vi "Variant to String.vi"(8 "error in (no error)":errorcluster, 10 "datatype":T1, 11 "Variant":variant) -> (0 "error out":errorcluster, 3 "String":string)   [LabVIEW 2016, in "DataGrid.lvlib" / "DataTable.lvclass"]
uses:
  <userlib>/LabVIEWdotNetDataGrid/source/DataTable/DataTable.lvclass
  <userlib>/LabVIEWdotNetDataGrid/source/GridColumn/ColumnType.ctl
  <userlib>/LabVIEWdotNetDataGrid/source/GridColumn/GridColumn.lvclass
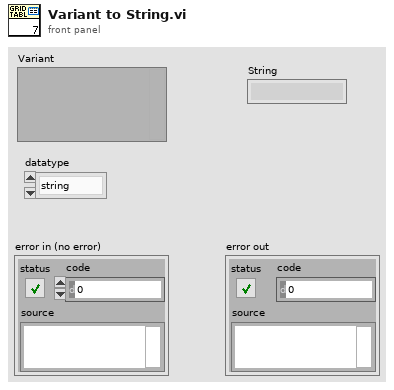
[diagram p1: front panel]
types:
  T1 = typedef "DataGrid.lvlib/GridColumn.lvclass/ColumnType.ctl" = enum16{"string", "image", "check", "numeric", "timestamp", "button", "combo", "link"}
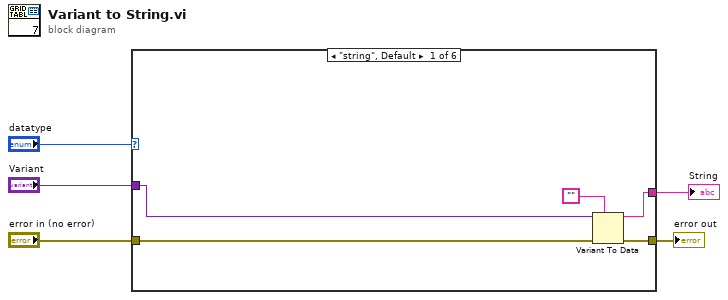
[diagram p0: block diagram]
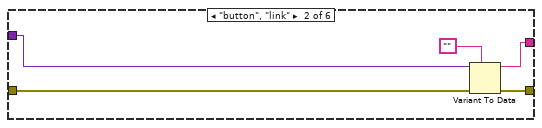
[diagram p2: hidden frame]
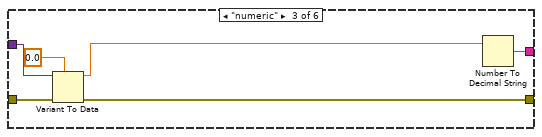
[diagram p3: hidden frame]
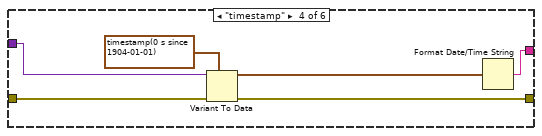
[diagram p4: hidden frame]
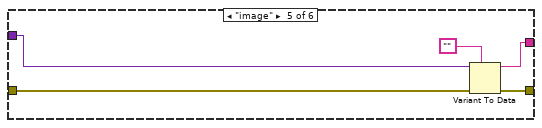
[diagram p5: hidden frame]
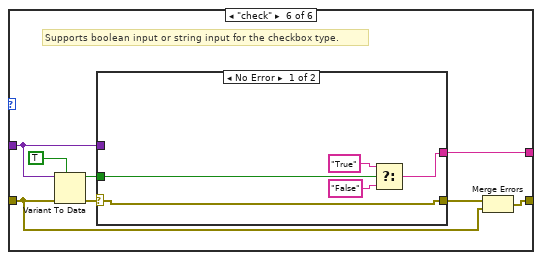
[diagram p6: hidden frame]
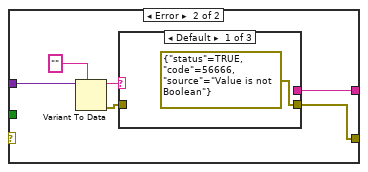
[diagram p7: hidden frame]
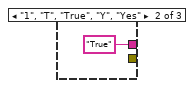
[diagram p8: hidden frame]
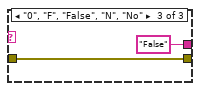
[diagram p9: hidden frame]
diagram:
  n1 = case shown="\"string\", Default" "datatype" {
    tunnel: "Variant" -> [w9 w14 w21 w27 w31 w37]
    tunnel: "error in (no error)" -> [w10 w15 w17 w23 w32 w35]
    tunnel: [w6 w11 w16 w22 w28 w34] -> w4
    tunnel: [w7 w12 w18 w24 w29 w33] -> w1
    frame "string", Default {
      n2 = Variant To Data(error in=w10, type="", Variant=w9) -> (data=w7:string, error out=w6:errorcluster)
    }
    frame "button", "link" {
      n3 = Variant To Data(error in=w15, type="", Variant=w14) -> (data=w12:string, error out=w11:errorcluster)
    }
    frame "numeric" {
      n4 = Variant To Data(error in=w17, type=0.0, Variant=w21) -> (data=w19:dbl, error out=w16:errorcluster)
      n5 = Number To Decimal String(number=w19) -> (decimal integer string=w18:string)  [unwired: 1 in]
    }
    frame "timestamp" {
      n6 = Variant To Data(error in=w23, type=timestamp(0 s since 1904-01-01), Variant=w27) -> (data=w25:timestamp, error out=w22:errorcluster)
      n7 = Format Date/Time String(seconds (now)=w25) -> (date/time string=w24:string)  [unwired: 2 in]
    }
    frame "image" {
      n8 = Variant To Data(error in=w32, type="", Variant=w31) -> (data=w29:string, error out=w28:errorcluster)
    }
    frame "check" {
      # "Supports boolean input or string input for the checkbox type."
      n9 = Variant To Data(error in=w35, type=TRUE, Variant=w37) -> (data=w38:bool, error out=w39:errorcluster)
      n10 = case shown="No Error" w39 {
        selector: w39 -> [w45 _]
        tunnel: [w45 w47] -> w36
        tunnel: w38 -> [w44 _]
        tunnel: w37 -> [_ w50]
        tunnel: [w41 w46] -> w33
        frame No Error {
          n11 = Select(t="True", s=w44, f="False") -> (s? t:f=w41:string)
        }
        frame Error {
          n12 = Variant To Data(type="", Variant=w50) -> (data=w51:string, error out=w48:errorcluster)  [unwired: 1 in]
          n13 = case shown="Default" w51 {
            tunnel: w48 -> [_ _ w55]
            tunnel: [errorcluster {"status"=TRUE, "code"=56666, "source"="Value is not Boolean"} ("error out") _ w55] -> w47
            tunnel: [_ "True" "False"] -> w46
            frame Default {
            }
            frame "1", "T", "True", "Y", "Yes" {
            }
            frame "0", "F", "False", "N", "No" {
            }
          }
        }
      }
      n14 = Merge Errors(w36, w35) -> (w34:errorcluster)
    }
  }
  "error out" <- w4
  "String" <- w1
